vi "Smoothed Graph.vi"(0 "Raw Graph":dbl[](array[numeric]), 1 "Times":u32[](array[numeric]), 3 "Averaging":string(combo)="30 s") -> (6 "Avg Graph":dbl[](array[numeric]), 7 "Mean":dbl, 8 "Last Value":dbl, 9 "Std. Dev.":dbl)   [LabVIEW 2009]
uses:
  <vilib>/Analysis/NI_AALBase.lvlib
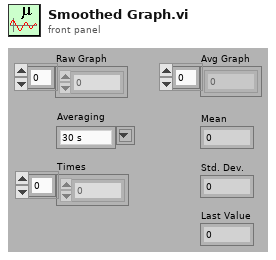
[diagram p1: front panel]
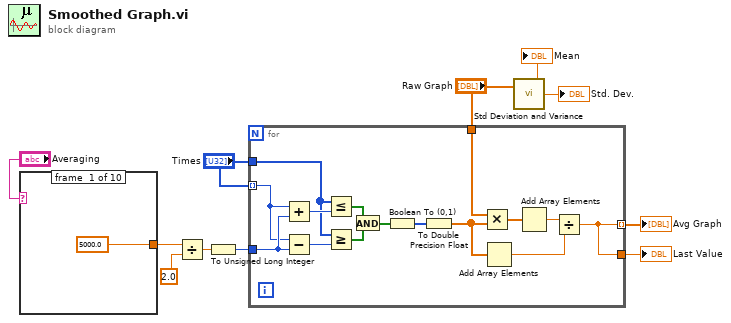
[diagram p0: block diagram]
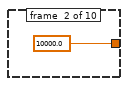
[diagram p2: hidden frame]
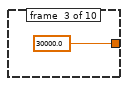
[diagram p3: hidden frame]
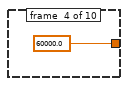
[diagram p4: hidden frame]
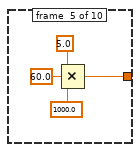
[diagram p5: hidden frame]
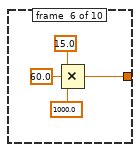
[diagram p6: hidden frame]
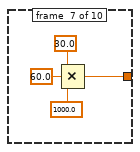
[diagram p7: hidden frame]
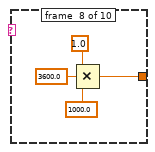
[diagram p8: hidden frame]
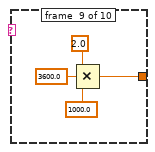
[diagram p9: hidden frame]
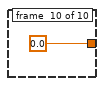
[diagram p10: hidden frame]
diagram:
  n1 = case shown="\"5 min\"" "Averaging" {
    tunnel: [5000.0 10000.0 30000.0 60000.0 w16 w20 w24 w28 w32 0.0] -> w10
    frame #0 {
    }
    frame #1 {
    }
    frame #2 {
    }
    frame #3 {
    }
    frame #4 {
      n2 = Compound Arithmetic op=MULTIPLY(5.0 ("value"), 60.0 ("value"), 1000.0 ("value")) -> (w16:dbl)
    }
    frame #5 {
      n3 = Compound Arithmetic op=MULTIPLY(15.0 ("value"), 60.0 ("value"), 1000.0 ("value")) -> (w20:dbl)
    }
    frame #6 {
      n4 = Compound Arithmetic op=MULTIPLY(30.0 ("value"), 60.0 ("value"), 1000.0 ("value")) -> (w24:dbl)
    }
    frame #7 {
      n5 = Compound Arithmetic op=MULTIPLY(1.0 ("value"), 3600.0 ("value"), 1000.0 ("value")) -> (w28:dbl)
    }
    frame #8 {
      n6 = Compound Arithmetic op=MULTIPLY(2.0 ("value"), 3600.0 ("value"), 1000.0 ("value")) -> (w32:dbl)
    }
    frame #9 {
    }
  }
  n7 = Divide(x=w10, y=2.0) -> (x/y=w7:dbl)
  n8 = To Unsigned Long Integer(number=w7) -> (unsigned 32bit integer=w6:u32)
  n9 = for {
    tunnel: "Times" -> [w50] mode=indexing
    tunnel: "Times" -> [w47]
    tunnel: w6 -> [w51]
    tunnel: "Raw Graph" -> [w42]
    tunnel: [w37] -> w5 mode=indexing
    tunnel: [w37] -> w2
    n10 = Add(x=w50, y=w51) -> (x+y=w48:u32)
    n11 = Subtract(x=w50, y=w51) -> (x-y=w49:u32)
    n12 = Less Or Equal?(x=w47, y=w48) -> (x <= y?=w46:bool[])
    n13 = Greater Or Equal?(x=w47, y=w49) -> (x >= y?=w45:bool[])
    n14 = And(x=w46, y=w45) -> (x .and. y?=w44:bool[])
    n15 = Boolean To (0,1)(Boolean=w44) -> (0, 1=w43:i16[])
    n16 = To Double Precision Float(number=w43) -> (double precision float=w38:dbl[])
    n17 = Multiply(x=w42, y=w38) -> (x*y=w39:dbl[])
    n18 = Add Array Elements(numeric array=w38) -> (sum=w41:dbl)
    n19 = Add Array Elements(numeric array=w39) -> (sum=w40:dbl)
    n20 = Divide(x=w40, y=w41) -> (x/y=w37:dbl)
  }
  "Avg Graph" <- w5
  "Last Value" <- w2
  n21 = call <vilib>:"Std Deviation and Variance.vi"("X"="Raw Graph") -> ("mean"=→"Mean":dbl, "standard deviation"=→"Std. Dev.":dbl)  [unwired: 1 in, 1 out]
